vi "Export Instrument Addon Configuration_ex.vi"() -> ()   [LabVIEW 2019]
uses:
  <vilib>/NI VeriStand/Custom Device API/Custom Device Item Ref.ctl
  Scripting API/Scripting API.lvlib
  <vilib>/NI VeriStand/Custom Device API/Custom Device API.lvlib
panel:
  out "Instrument Addon Refnum Out":T1=18446744073709551615 format="%.0x"
  out "Error Out":errorcluster
  in  "Instrument Addon Refnum In":T1=18446744073709551615 format="%.0x"
  in  "Exported File Path":path
  in  "Error In":errorcluster
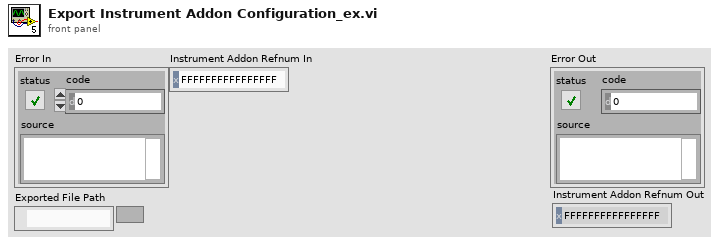
[diagram p1: front panel]
types:
  T1 = typedef "Custom Device API.lvlib/Custom Device Item Ref.ctl" = u64
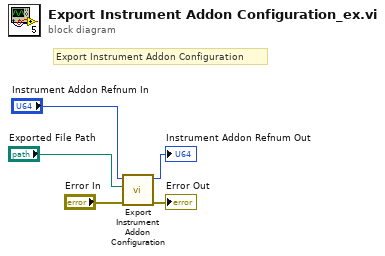
[diagram p0: block diagram]
diagram:
  # "Export Instrument Addon Configuration"
  n1 = call "Export Instrument Addon Configuration.vi"("Error In"="Error In", "Exported File Path"="Exported File Path", "Instrument Addon Refnum In"="Instrument Addon Refnum In") -> ("Error Out"=→"Error Out":errorcluster, "Instrument Addon Refnum Out"=→"Instrument Addon Refnum Out":T1)  [unwired: 7 in]
